vi "ChapR cRIO Translater.vi"(6 "Position":u8=49, 7 "CMD":u8, 8 "Alliance":u8=66, 10 "ChapR Data":string, 11 "TeamNo":u16) -> (2 "Network Data":string)   [LabVIEW 2013]
uses:
  ChapR Packet.ctl
  Driver Station Packet.ctl
panel:
  out "value":T1
  in  "Network Packet 2":T1
  in  "Network Packet":T1
  in  "ChapR Packet":T2
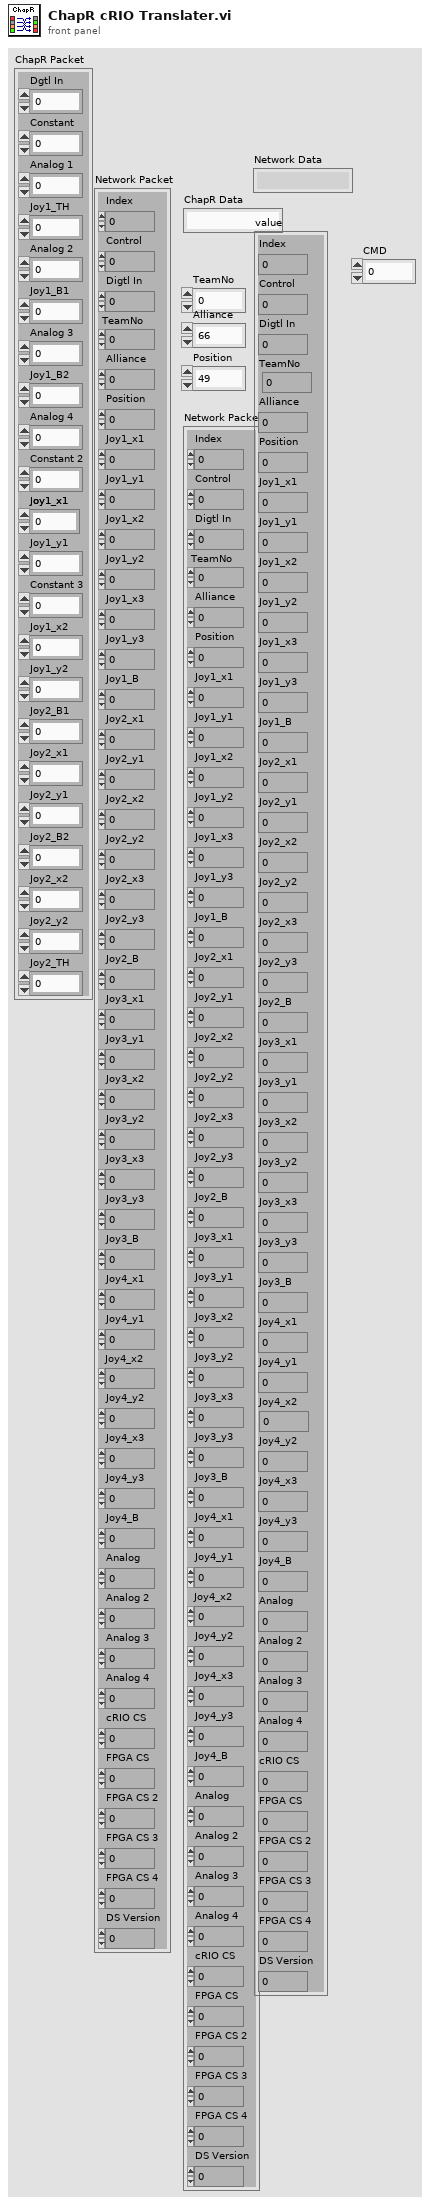
[diagram p1: front panel]
types:
  T1 = typedef "Driver Station Packet.ctl" = cluster{"Index":u16, "Control":u8, "Digtl In":u8, "TeamNo":u16, "Alliance":u8, "Position":u8, "Joy1_x1":i8, "Joy1_y1":i8, "Joy1_x2":i8, "Joy1_y2":i8, "Joy1_x3":i8, "Joy1_y3":i8, "Joy1_B":u16, "Joy2_x1":i8, "Joy2_y1":i8, "Joy2_x2":i8, "Joy2_y2":i8, "Joy2_x3":i8, "Joy2_y3":i8, "Joy2_B":u16, "Joy3_x1":i8, "Joy3_y1":i8, "Joy3_x2":i8, "Joy3_y2":i8, "Joy3_x3":i8, "Joy3_y3":i8, "Joy3_B":u16, "Joy4_x1":i8, "Joy4_y1":i8, "Joy4_x2":i8, "Joy4_y2":i8, "Joy4_x3 ":i8, "Joy4_y3":i8, "Joy4_B":u16, "Analog":u16, "Analog 2":u16, "Analog 3":u16, "Analog 4":u16, "cRIO CS":u64, "FPGA CS":u32, "FPGA CS 2":u32, "FPGA CS 3":u32, "FPGA CS 4":u32, "DS Version":u64}
  T2 = typedef "ChapR Packet.ctl" = cluster{"Dgtl In":u8, "Constant":u8, "Analog 1":u16, "Joy1_TH":u8, "Analog 2":u16, "Joy1_B1":u8, "Analog 3":u16, "Joy1_B2":u8, "Analog 4":u16, "Constant 2":u8, "Joy1_x1":i8, "Joy1_y1":i8, "Constant 3":u8, "Joy1_x2":i8, "Joy1_y2":i8, "Joy2_B1":u8, "Joy2_x1":i8, "Joy2_y1":i8, "Joy2_B2":u8, "Joy2_x2":i8, "Joy2_y2":i8, "Joy2_TH":u8}
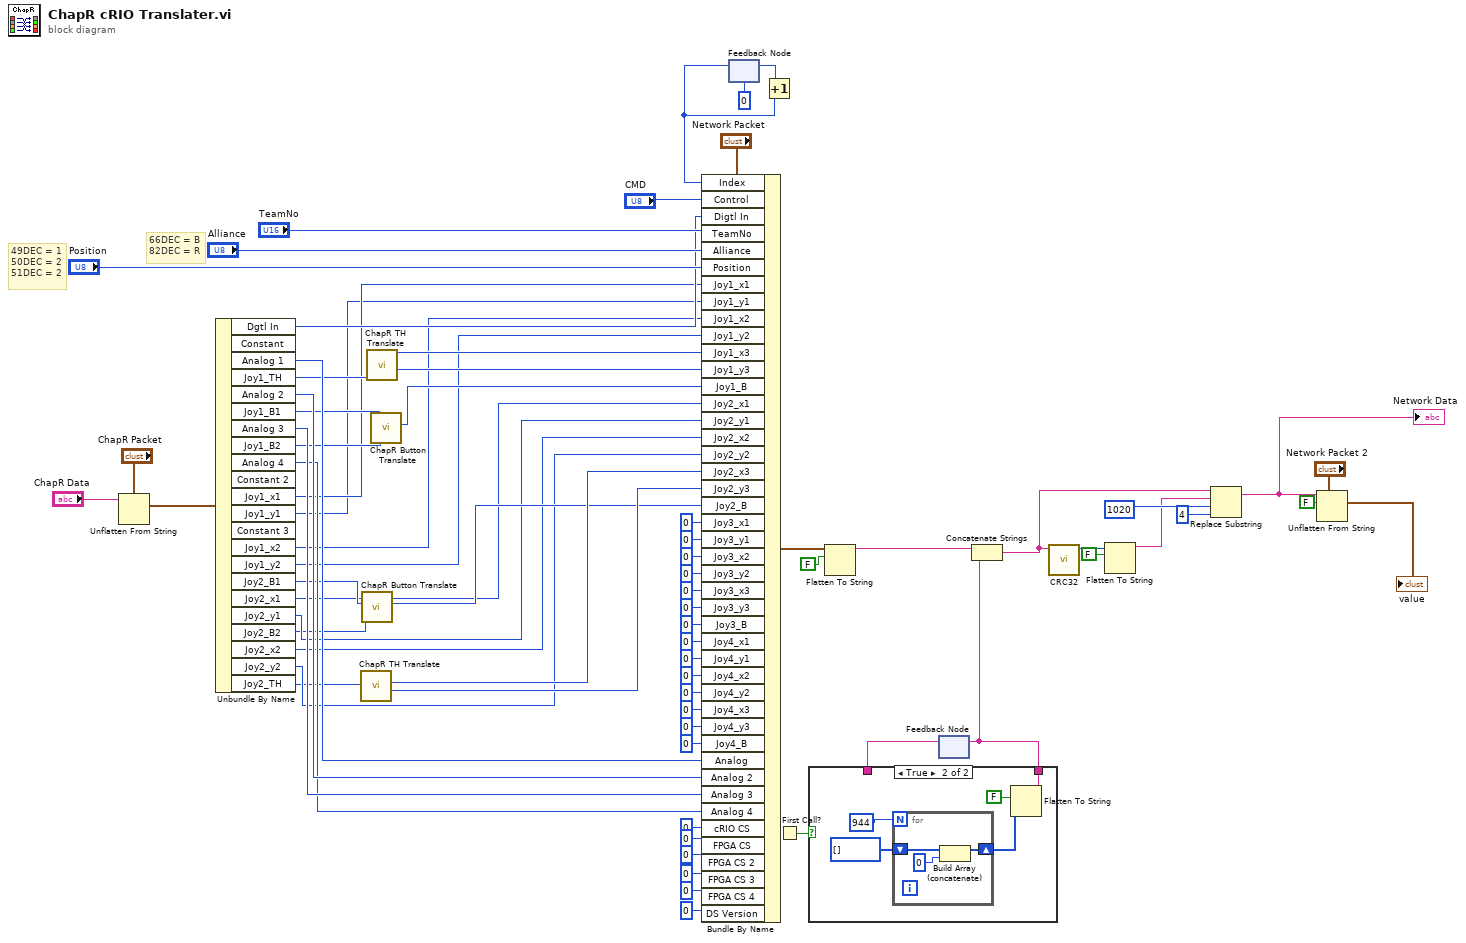
[diagram p0: block diagram]
diagram:
  # "49DEC = 1\n50DEC = 2\n51DEC = 2"
  # "66DEC = B\n82DEC = R"
  n1 = Unflatten From String(type="ChapR Packet", binary string="ChapR Data") -> (value=w70:T2)  [unwired: 3 in, 2 out]
  n2 = Unbundle By Name(w70) -> ("Dgtl In"=w19:u8, "Analog 1"=w18:u16, "Joy1_TH"=w17:u8, "Analog 2"=w16:u16, "Joy1_B1"=w15:u8, "Analog 3"=w14:u16, "Joy1_B2"=w13:u8, "Analog 4"=w12:u16, "Joy1_x1"=w11:i8, "Joy1_y1"=w10:i8, "Joy1_x2"=w9:i8, "Joy1_y2"=w8:i8, "Joy2_B1"=w7:u8, "Joy2_x1"=w1:i8, "Joy2_y1"=w6:i8, "Joy2_B2"=w5:u8, "Joy2_x2"=w4:i8, "Joy2_y2"=w3:i8, "Joy2_TH"=w2:u8)  [unwired: 3 out]
  n3 = call "ChapR TH Translate.vi"("Tophat Value"=w2) -> ("Y"=w65:i8, "X"=w64:i8)  [unwired: 9 in]
  n4 = call "ChapR Button Translate.vi"("B2"=w5, "B1"=w7) -> ("B"=w42:u16)  [unwired: 9 in]
  n5 = call "ChapR TH Translate.vi"("Tophat Value"=w17) -> ("Y"=w66:i8, "X"=w67:i8)  [unwired: 9 in]
  n6 = call "ChapR Button Translate.vi"("B2"=w13, "B1"=w15) -> ("B"=w63:u16)  [unwired: 9 in]
  n7 = feedback #1(u16 0) -> (w40:u16)
  n8 = Bundle By Name(cluster="Network Packet", "Index"=w40, "Control"="CMD", "Digtl In"=w19, "TeamNo"="TeamNo", "Alliance"="Alliance", "Position"="Position", "Joy1_x1"=w11, "Joy1_y1"=w10, "Joy1_x2"=w9, "Joy1_y2"=w8, "Joy1_x3"=w67, "Joy1_y3"=w66, "Joy1_B"=w63, "Joy2_x1"=w1, "Joy2_y1"=w6, "Joy2_x2"=w4, "Joy2_y2"=w3, "Joy2_x3"=w64, "Joy2_y3"=w65, "Joy2_B"=w42, "Joy3_x1"=i8 0, "Joy3_y1"=i8 0, "Joy3_x2"=i8 0, "Joy3_y2"=i8 0, "Joy3_x3"=i8 0, "Joy3_y3"=i8 0, "Joy3_B"=u16 0, "Joy4_x1"=i8 0, "Joy4_y1"=i8 0, "Joy4_x2"=i8 0, "Joy4_y2"=i8 0, "Joy4_x3"=i8 0, "Joy4_y3"=i8 0, "Joy4_B"=u16 0, "Analog"=w18, "Analog 2"=w16, "Analog 3"=w14, "Analog 4"=w12, "cRIO CS"=u64 0, "FPGA CS"=u32 0, "FPGA CS 2"=u32 0, "FPGA CS 3"=u32 0, "FPGA CS 4"=u32 0, "DS Version"=u64 0) -> (w69:T1)
  n9 = Increment(x=w40) -> (x+1=w39:u16)
  n10 = feedback-in #1(w39) -> ()
  n11 = First Call?() -> (First Call?: T/F=w26:bool)
  n12 = Flatten To String(anything=w69, prepend array or string size? (T)=FALSE) -> (data string=w23:string)  [unwired: 2 in, 2 out]
  n13 = feedback #2() -> (w25:string)  [unwired: 1 in]
  n14 = case shown="True" w26 {
    tunnel: [w73 w75] -> w22
    tunnel: w25 -> [w73 _]
    frame False {
    }
    frame True {
      n15 = for {
        N: 944 -> [_]
        shift-right: [w79] -> w76
        shift-left: u8[] [] -> [w81]
        n16 = Build Array (concatenate)(w81, u8 0) -> (w79:u8[])
      }
      n17 = Flatten To String(anything=w76, prepend array or string size? (T)=FALSE) -> (data string=w75:string)  [unwired: 2 in, 2 out]
    }
  }
  n18 = feedback-in #2(w22) -> ()
  n19 = Concatenate Strings(w23, w22) -> (w24:string)
  n20 = call "CRC32.vi"("Data"=w24) -> ("CRC32Value"=w33:u32)  [unwired: 10 in]
  n21 = Flatten To String(anything=w33, prepend array or string size? (T)=FALSE) -> (data string=w32:string)  [unwired: 2 in, 2 out]
  n22 = Replace Substring(2:4 ("length (len. of substring)"), 3:1020 ("offset (0)"), 4:w32, 5:w24) -> (1:w21:string)  [unwired: 1 out]
  "Network Data" <- w21
  n23 = Unflatten From String(type="Network Packet 2", binary string=w21, data includes array or string size? (T)=FALSE) -> (value=→"value":T1)  [unwired: 2 in, 2 out]
